vi "MGI Handler Wrapper.vi"(9 "Ignore Warn?":bool, 10 "Log Directory":path, 11 "Error Reporter":refnum<class "MGI Error Reporter Base.lvclass">) -> ()   [LabVIEW 2020, in "MGI Error Reporter Base.lvclass"]
doc: "Wrapper for the daemon. This VI exists so that a non-dynamic dispatch VI may be run dynamically in a separate exectution thread. The actual daemon used is the Loop.vi of the specified Error Reporter class.\n\nAuthored by Shawn Walpole\nsupport@mooregoodideas.com\nwww.mooregoodideas.com\n\nCopyright (c) 2010, Moore Good Ideas, Inc.\n\nAll rights reserved.\n\nRedistribution and use in source and binary forms, with or without modification, are permitted provided that the following conditions are met:\n\n * Redistributions of source code must retain the above copyright notice, this list of conditions and the following disclaimer.\n * Redistributions in binary form must reproduce the above copyright notice, this list of conditions and the following disclaimer in the documentation and/or other materials provided with the distribution.\n * Neither the name of Moore Good Ideas, Inc. nor the names of its contributors may be used to endorse or promote products derived from this software without specific prior written permission.\n\nTHIS SOFTWARE IS PROVIDED BY THE COPYRIGHT HOLDERS AND CONTRIBUTORS \"AS IS\" AND ANY EXPRESS OR IMPLIED WARRANTIES, INCLUDING, BUT NOT LIMITED TO, THE IMPLIED WARRANTIES OF MERCHANTABILITY AND FITNESS FOR A PARTICULAR PURPOSE ARE DISCLAIMED. IN NO EVENT SHALL THE COPYRIGHT OWNER OR CONTRIBUTORS BE LIABLE FOR ANY DIRECT, INDIRECT, INCIDENTAL, SPECIAL, EXEMPLARY, OR CONSEQUENTIAL DAMAGES (INCLUDING, BUT NOT LIMITED TO, PROCUREMENT OF SUBSTITUTE GOODS OR SERVICES; LOSS OF USE, DATA, OR PROFITS; OR BUSINESS INTERRUPTION) HOWEVER CAUSED AND ON ANY THEORY OF LIABILITY, WHETHER IN CONTRACT, STRICT LIABILITY, OR TORT (INCLUDING NEGLIGENCE OR OTHERWISE) ARISING IN ANY WAY OUT OF THE USE OF THIS SOFTWARE, EVEN IF ADVISED OF THE POSSIBILITY OF SUCH DAMAGE."
uses:
  <userlib>/_MGI/Error Reporter/MGI Error Reporter Base/MGI Error Reporter Base.lvclass
  <userlib>/_MGI/Error Reporter/MGI Error Reporter Base/Protected/MGI Cmd Enum.ctl
  <userlib>/_MGI/Error Reporter/MGI Error Reporter Base/Private/MGI Globals.vi
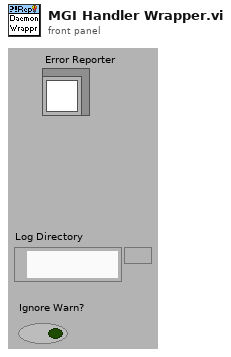
[diagram p1: front panel]
types:
  T1 = typedef "MGI Error Reporter Base.lvclass/MGI Cmd Enum.ctl" = enum16{"Quit", "Show UI"}
  T2 = typedef "MGI Error Reporter Base.lvclass/Cmd Enum.ctl" = enum16{"Quit", "Show UI"}
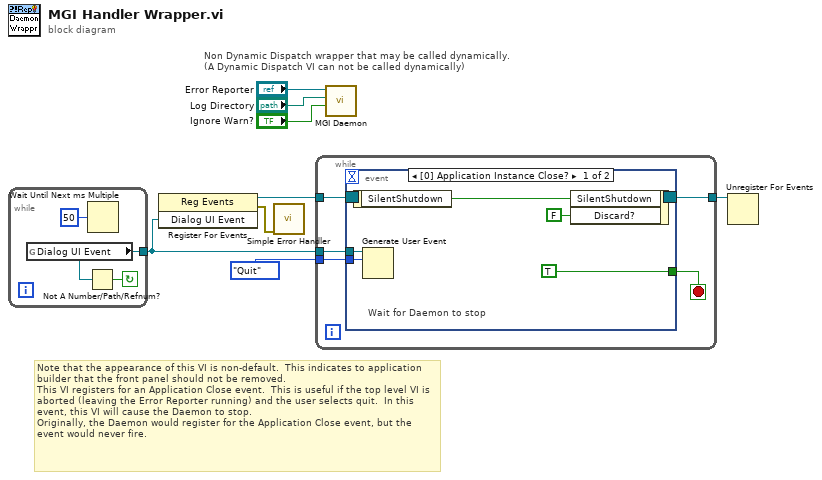
[diagram p0: block diagram]
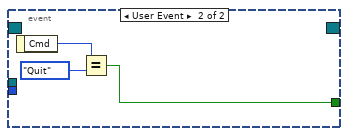
[diagram p2: hidden frame]
diagram:
  # "Note that the appearance of this VI is non-default.  This indicates to application builder that the front panel should not be removed.\nThis VI registers for an Application Close event.  This is useful if the top level VI is aborted (leaving the Error Reporter running) and the user selects quit.  In this event, this VI will cause the Daemon to stop.\nOriginally, the Daemon would register for the Application Close event, but the event would never fire."
  # "Non Dynamic Dispatch wrapper that may be called dynamically.\n(A Dynamic Dispatch VI can not be called dynamically)"
  n1 = while {
    tunnel: [w9] -> w3
    stop <- w11 continue-if-true
    n2 = global read "MGI Globals.vi" "Dialog UI Event"() -> (w9:refnum<user-event>)
    n3 = Not A Number/Path/Refnum?(number/path/refnum=w9) -> (NaN/Path/Refnum?=w11:bool)
    n4 = Wait Until Next ms Multiple(millisecond multiple=u32 50) -> ()  [unwired: 1 out]
  }
  n5 = register-events(w3) -> (reference out=w4:refnum<event-registration>, error out=w5:errorcluster)  [unwired: 2 in]
  n6 = call <vilib>:"Simple Error Handler.vi"("error in (no error)"=w5) -> ()  [unwired: 1 in, 8 out]
  n7 = while {
    tunnel: w4 -> [w16]
    tunnel: w3 -> [w15]
    tunnel: MGI_Cmd_Enum."Quit" ("event data") -> [w13]
    tunnel: [w12] -> w1
    stop <- w14 stop-if-true
    n8 = event shown="[0] Application Instance Close?" {
      selector: w16 -> [_ _]
      dyn-events: [_ _] -> w12
      timeout: _ -> [_ _]
      tunnel: w15 -> [w21 _]
      tunnel: [TRUE ("Discard?") w22] -> w14
      tunnel: w13 -> [w20 _]
      event Application Instance Close? {
        # "Wait for Daemon to stop"
        n9 = event-data() -> ("SilentShutdown"=w18:bool)  [unwired: 1 out]
        n10 = Generate User Event(user event=w21, event data cluster=w20) -> ()  [unwired: 2 in, 2 out]
        n11 = event-data("SilentShutdown"=w18, "Discard?"=FALSE) -> ()  [unwired: 1 in, 1 out]
      }
      event User Event {
        n12 = event-data() -> ("Cmd"=w24:T2)  [unwired: 1 out]
        n13 = Equal?(x=w24, y=MGI_Cmd_Enum."Quit") -> (x = y?=w22:bool)
      }
    }
  }
  n14 = call-dynamic "MGI Daemon.vi"("Ignore Warnings? (F: Process Errors and Warnings)"="Ignore Warn?", "Error Log Directory"="Log Directory", "MGI Error Reporter Base In"="Error Reporter") -> ()  [unwired: 9 out]
  n15 = Unregister For Events(event registration refnum=w1) -> ()  [unwired: 1 in, 1 out]
